vi "Headers.vi"(8 "error in (no error)":errorcluster, 11 "LabVIEW Web Service Request":refnum<class "Web Request.lvclass">) -> (0 "error out":errorcluster, 3 "LabVIEW Web Service Request out":refnum<class "Web Request.lvclass">)   [LabVIEW 2014]
doc: "Sets all required headers by the SSE connection"
uses:
  <vilib>/wsapi/Web Request.lvclass
  Configuration/Global_Configurations.vi
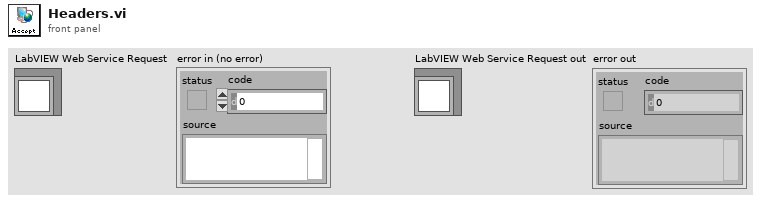
[diagram p1: front panel]
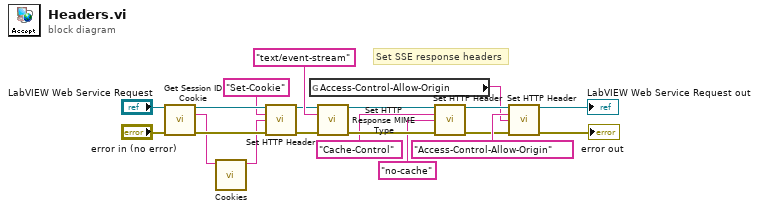
[diagram p0: block diagram]
diagram:
  # "Set SSE response headers"
  n1 = call <vilib>:"Get Session ID Cookie.vi"("LabVIEW Web Service Request"="LabVIEW Web Service Request", "error in (no error)"="error in (no error)") -> ("LabVIEW Web Service Request out"=w11:refnum<class "Web Request.lvclass">, "session ID cookie"=w5:string, "error out"=w12:errorcluster)  [unwired: 11 in]
  n2 = call "Cookies.vi"("ID cookie"=w5) -> ("cookie header"=w10:string)  [unwired: 10 in]
  n3 = call <vilib>:"Set HTTP Header.vi"("LabVIEW Web Service Request"=w11, "header"="Set-Cookie", "header value"=w10, "error in (no error)"=w12) -> ("LabVIEW Web Service Request out"=w8:refnum<class "Web Request.lvclass">, "error out"=w7:errorcluster)  [unwired: 10 in]
  n4 = global read "Global_Configurations.vi" "Access-Control-Allow-Origin"() -> (w13:string)
  n5 = call <vilib>:"Set HTTP Response MIME Type.vi"("LabVIEW Web Service Request"=w8, "MIME type (text/html)"="text/event-stream" ("header"), "error in (no error)"=w7) -> ("LabVIEW Web Service Request out"=w20:refnum<class "Web Request.lvclass">, "error out"=w19:errorcluster)  [unwired: 11 in]
  n6 = call <vilib>:"Set HTTP Header.vi"("LabVIEW Web Service Request"=w20, "header"="Cache-Control", "header value"="no-cache", "error in (no error)"=w19) -> ("LabVIEW Web Service Request out"=w16:refnum<class "Web Request.lvclass">, "error out"=w15:errorcluster)  [unwired: 10 in]
  n7 = call <vilib>:"Set HTTP Header.vi"("LabVIEW Web Service Request"=w16, "header"="Access-Control-Allow-Origin", "header value"=w13, "error in (no error)"=w15) -> ("LabVIEW Web Service Request out"=→"LabVIEW Web Service Request out":refnum<class "Web Request.lvclass">, "error out"=→"error out":errorcluster)  [unwired: 10 in]
